vi "design info to var.vi"(10 "Design Inputs":T2={"Q.Plant"=0.005, "C.CoagDoseMax"=0.01, "C.CoagStock"=0.015, "Ti.CoagStock"=0.0015, "EN.DrillSeries"=enum."English", "EN.TubeSeries"=enum."English", "N.SedTanks"=10.0, "N.SedBaysEst"=240.0, "W.SedPlate"=0.02, "L.SedPlateSheet"=0.0, "T.SedPlate"=388800000.0, "T.PlantWall"=0.03, "H.FlocOption"=0.01, "T.FlocBaffleRigidH"=0.03, "T.ConcreteMin"=0.3, "T.SedWeir"=0.3, "T.FlocBaffleRigidV"=108000.0} {"T.FlocBaffleRigidV" min=0.0 max=0.2 step=0.001 format="%#.1f"; "T.SedWeir" min=0.001 max=0.2 step=0.001 format="%#.1f"; "T.SedPlate" min=0.001 max=0.05 step=0.001 format="%#.1f"; "T.FlocBaffleRigidH" min=0.0 max=0.2 step=0.001 format="%#.1f"; "T.ConcreteMin" min=0.005 max=0.2 step=0.001 format="%#.1f"; "L.SedPlateSheet" min=0.3 max=8.0 step=0.01 format="%#.1f"; "N.SedBaysEst" min=1.0 max=20.0 step=1.0 format="%#.0f"; "N.SedTanks" min=1.0 max=20.0 step=1.0 format="%#.0f"; "Ti.CoagStock" min=43200.0 max=360000.0 step=3600.0 format="%#.1f"; "H.FlocOption" min=0.5 max=4.0 step=0.01 format="%#.2f"; "C.CoagStock" min=50.0 max=500.0 step=1.0 format="%#.0f"; "C.CoagDoseMax" min=0.03 max=0.2 step=0.005 format="%#.0f"; "Q.Plant" min=0.001 max=0.2 step=0.0001 format="%#.1f"; "T.PlantWall" min=0.05 max=0.5 step=0.001 format="%#.1f"; "W.SedPlate" min=0.5 max=3.0 step=0.001 format="%#.1f"}, 11 "Project Info":T1) -> (3 "Array to save":cluster{"Label.Text":string, "Value":variant}[](array[cluster]))   [LabVIEW 2015]
uses:
  Basic Inputs.ctl
  Project inputs.ctl
  AguaClara Library.lvlib
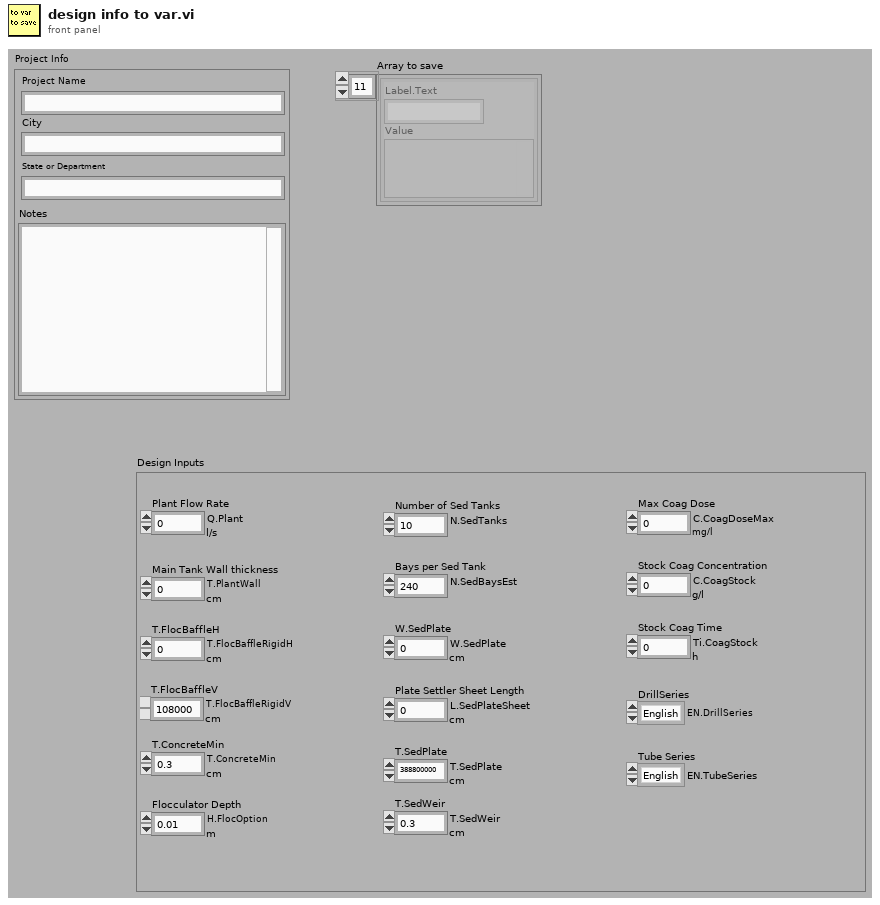
[diagram p1: front panel]
types:
  T1 = typedef "AguaClara Library.lvlib/Project inputs.ctl" = cluster{"Project Name":string, "City":string, "State":string, "Notes":string}
  T2 = typedef "AguaClara Library.lvlib/Basic Inputs.ctl" = cluster{"Q.Plant":dbl[unit], "C.CoagDoseMax":dbl[unit], "C.CoagStock":dbl[unit], "Ti.CoagStock":dbl[unit], "EN.DrillSeries":enum16{"English", "Metric"}, "EN.TubeSeries":enum16{"English", "Metric"}, "N.SedTanks":dbl, "N.SedBaysEst":dbl, "W.SedPlate":dbl[unit], "L.SedPlateSheet":dbl[unit], "T.SedPlate":dbl[unit], "T.PlantWall":dbl[unit], "H.FlocOption":dbl[unit], "T.FlocBaffleRigidH":dbl[unit], "T.ConcreteMin":dbl[unit], "T.SedWeir":dbl[unit], "T.FlocBaffleRigidV":dbl[unit]}
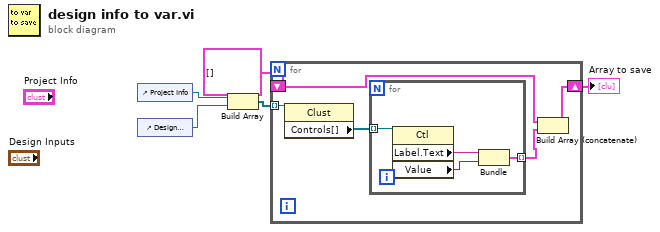
[diagram p0: block diagram]
diagram:
  n1 = control-ref of="Project Info"() -> (w5:refnum<vi>)
  n2 = control-ref of="Design Inputs"() -> (w4:refnum<vi>)
  n3 = Build Array(w5, w4) -> (w3:refnum<vi>[])
  n4 = for {
    tunnel: w3 -> [w10] mode=indexing
    shift-right: [w6] -> w2
    shift-left: cluster{"Label.Text":string, "Value":variant}[] [] -> [w7]
    n5 = property class="Clust"(reference=w10) -> ("Controls[]"=w9:refnum<vi>[])  [unwired: 1 in, 2 out]
    n6 = for {
      tunnel: w9 -> [w14] mode=indexing
      tunnel: [w11] -> w8 mode=indexing
      n7 = property class="Ctl"(reference=w14) -> ("Label.Text"=w13:string, "Value"=w12:variant)  [unwired: 1 in, 2 out]
      n8 = Bundle("Label.Text"=w13, "Value"=w12) -> (w11:cluster{"Label.Text":string, "Value":variant})  [unwired: 1 in]
    }
    n9 = Build Array (concatenate)(w7, w8) -> (w6:cluster{"Label.Text":string, "Value":variant}[])
  }
  "Array to save" <- w2
